vi "Stop Core.vi"(10 "final error code":i32, 11 "cRIO-CO2 in":refnum<class "cRIO-CO2.lvclass">) -> (3 "cRIO-CO2 out":refnum<class "cRIO-CO2.lvclass">)   [LabVIEW 2015, in "cRIO-Carbondioxide.lvlib" / "cRIO-CO2.lvlib" / "cRIO-CO2.lvclass"]
doc: "(<B>Filename</B>: Actor Framework.lvlib:Actor.lvclass:Stop Core.vi)\n\nDefines what the actor does before it stops. Use the <B>final error code</B> input to determine whether the actor shut down in response to an error.\n\nBy default, this method does nothing. A descendant class may override it to define behavior, such as shutting down any processes the actor initiated in its override of the Actor Core method."
uses:
  cRIO-CO2.lvclass
  cRIO-CO2.lvclass/cRIO-CO2.ctl
  <vilib>/ActorFramework/Time-Delayed Send Message/Time-Delay Override Options.ctl
  <vilib>/ActorFramework/Actor/Actor.lvclass
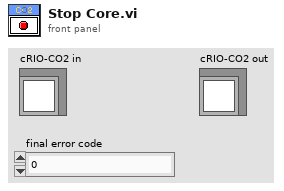
[diagram p1: front panel]
types:
  T1 = typedef "Time-Delay Override Options.ctl" = enum16{"Send next copy now", "Skip next scheduled copy", "Send next copy now and stop all further copies", "Stop all further copies"}
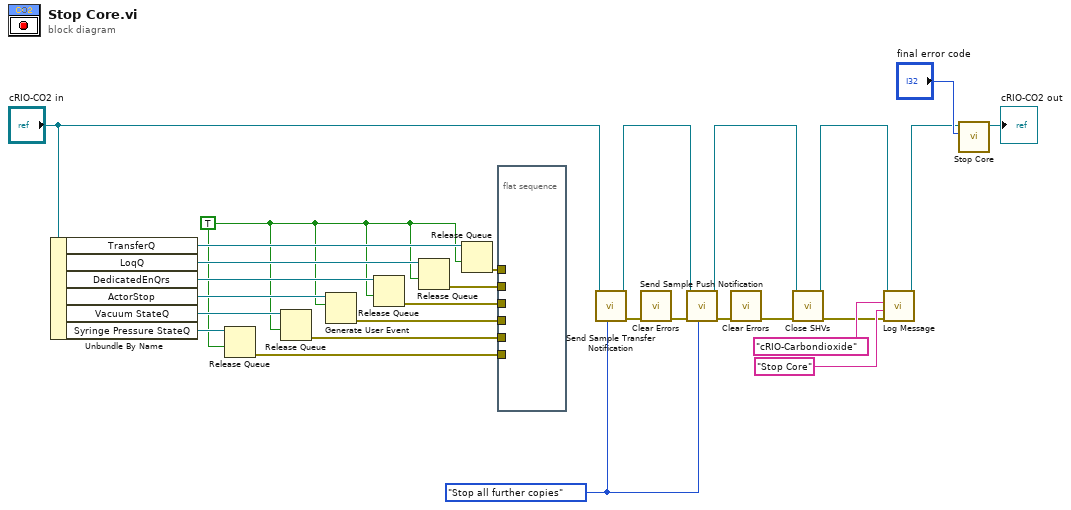
[diagram p0: block diagram]
diagram:
  w12 = Time-Delay_Override_Options."Stop all further copies" ("notification (Send next copy now)")
  w2 = TRUE ("event data")
  n1 = Unbundle By Name("cRIO-CO2 in") -> ("TransferQ"=w7:refnum<queue>, "LoqQ"=w20:refnum<queue>, "DedicatedEnQrs"=w21:refnum<queue>, "ActorStop"=w11:refnum<user-event>, "Vacuum StateQ"=w5:refnum<queue>, "Syringe Pressure StateQ"=w3:refnum<queue>)
  n2 = Release Queue(queue=w3, force destroy? (F)=w2) -> (error out=w1:errorcluster)  [unwired: 1 in, 2 out]
  n3 = Release Queue(queue=w5, force destroy? (F)=w2) -> (error out=w4:errorcluster)  [unwired: 1 in, 2 out]
  n4 = Generate User Event(user event=w11, event data cluster=w2) -> (error out=w10:errorcluster)  [unwired: 2 in, 1 out]
  n5 = Release Queue(queue=w21, force destroy? (F)=w2) -> (error out=w9:errorcluster)  [unwired: 1 in, 2 out]
  n6 = Release Queue(queue=w20, force destroy? (F)=w2) -> (error out=w8:errorcluster)  [unwired: 1 in, 2 out]
  n7 = Release Queue(queue=w7, force destroy? (F)=w2) -> (error out=w6:errorcluster)  [unwired: 1 in, 2 out]
  n8 = flat-sequence {
    tunnel: w10 -> [_]
    tunnel: w9 -> [_]
    tunnel: w8 -> [_]
    tunnel: w6 -> [_]
    tunnel: w4 -> [_]
    tunnel: w1 -> [_]
    frame #0 {
    }
  }
  n9 = call "Send Sample Transfer Notification.vi"("notification (Send next copy now)"=w12, "cRIO-CO2 in"="cRIO-CO2 in") -> ("error out"=w18:errorcluster, "cRIO-CO2 out"=w14:refnum<class "cRIO-CO2.lvclass">)  [unwired: 8 in]
  n10 = call <vilib>:"Clear Errors.vi"("error in (no error)"=w18) -> ("error out"=w17:errorcluster)  [unwired: 5 in, 1 out]
  n11 = call "Send Sample Push Notification.vi"("notification (Send next copy now)"=w12, "error in (no error)"=w17, "cRIO-CO2 in"=w14) -> ("error out"=w16:errorcluster, "cRIO-CO2 out"=w13:refnum<class "cRIO-CO2.lvclass">)  [unwired: 7 in]
  n12 = call <vilib>:"Clear Errors.vi"("error in (no error)"=w16) -> ("error out"=w15:errorcluster)  [unwired: 5 in, 1 out]
  n13 = call "Close SHVs.vi"("error in (no error)"=w15, "cRIO-CO2 in"=w13) -> ("error out"=w24:errorcluster, "cRIO-CO2 out"=w23:refnum<class "cRIO-CO2.lvclass">)  [unwired: 8 in]
  n14 = call "Log Message.vi"("error in (no error)"=w24, "String"="Stop Core", "Source Name"="cRIO-Carbondioxide", "cRIO-CO2 in"=w23) -> ("cRIO-CO2 out"=w22:refnum<class "cRIO-CO2.lvclass">)  [unwired: 6 in, 1 out]
  n15 = call-parent "Stop Core.vi"("final error code"="final error code", "Actor in"=w22) -> ("Actor out"=→"cRIO-CO2 out":refnum<class "cRIO-CO2.lvclass">)  [unwired: 9 in]
